vi "for循环的各种应用.vi"() -> ()   [LabVIEW 2019]
panel:
  out "索引 3":dbl[](array[numeric])
  out "索引 2":dbl[](array[numeric])
  out "索引":dbl[](array[numeric])
  out "上一次随机数":dbl
  out "最新的随机数":dbl
  out "循环计数端":i32
  in  "循环总数":i32
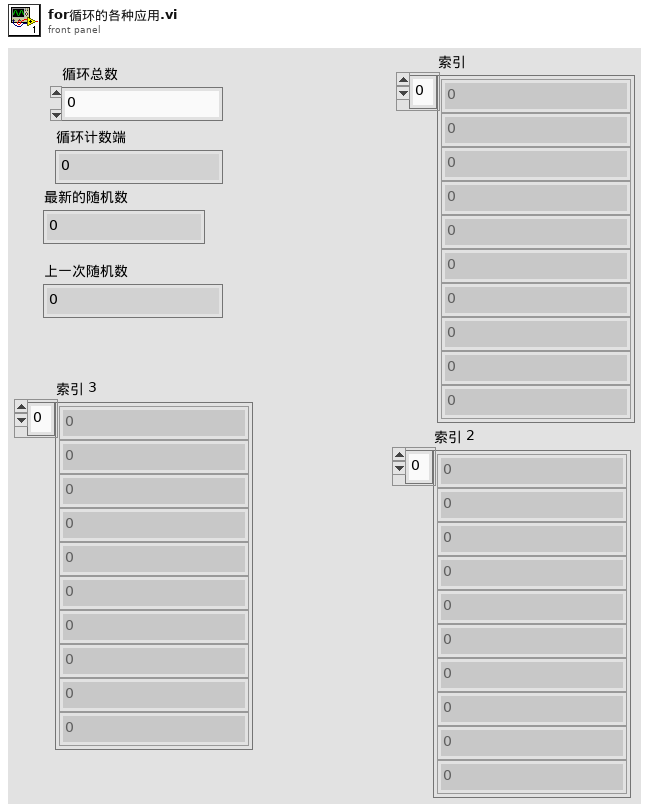
[diagram p1: front panel]
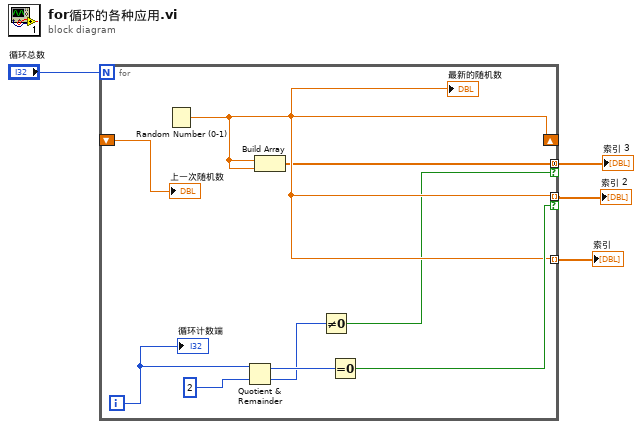
[diagram p0: block diagram]
diagram:
  n1 = for {
    N: "循环总数" -> [_]
    shift-right: [w8] -> _
    shift-left: _ -> [w13]
    tunnel: [w8] -> w3 mode=indexing
    tunnel: [w8] -> w2 mode=indexing if=w9
    tunnel: [w7] -> w1 mode=concatenating if=w6
    i -> [w11]
    n2 = Random Number (0-1)() -> (number: 0 to 1=w8:dbl)
    "最新的随机数" <- w8
    n3 = Quotient & Remainder(x=w11, y=2) -> (x-y*floor(x/y)=w10:i32, floor(x/y)=w5:i32)
    n4 = Build Array(w8, w8) -> (w7:dbl[])
    n5 = Not Equal To 0?(x=w5) -> (x != 0?=w6:bool)
    n6 = Equal To 0?(x=w10) -> (x = 0?=w9:bool)
    "循环计数端" <- w11
    "上一次随机数" <- w13
  }
  "索引" <- w3
  "索引 2" <- w2
  "索引 3" <- w1
